vi "next order.vi"(8 "error in":errorcluster, 10 "Order":string, 11 "status":T1) -> (0 "error out":errorcluster, 3 "Order":string)   [LabVIEW 2015]
uses:
  status.ctl
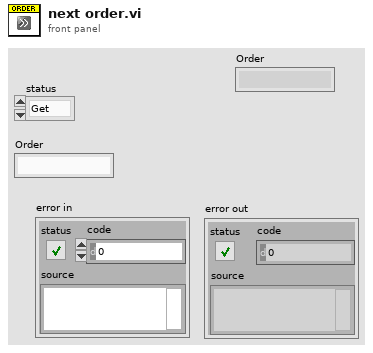
[diagram p1: front panel]
types:
  T1 = typedef "status.ctl" = enum16{"Get", "Set"}
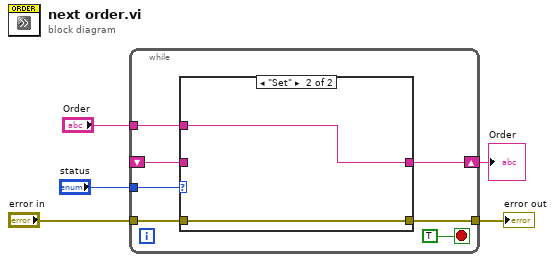
[diagram p0: block diagram]
diagram:
  n1 = while {
    shift-right: [w10] -> w1
    shift-left: _ -> [w8]
    tunnel: "status" -> [w11]
    tunnel: "Order" -> [w9]
    tunnel: "error in" -> [w7]
    tunnel: [w6] -> w2
    stop <- TRUE stop-if-true
    n2 = case shown="\"Set\"" w11 {
      tunnel: [w14 w16] -> w10
      tunnel: w9 -> [_ w16]
      tunnel: w8 -> [w14 _]
      tunnel: w7 -> [w13 w15]
      tunnel: [w13 w15] -> w6
      frame "Get", Default {
      }
      frame "Set" {
      }
    }
  }
  "error out" <- w2
  "Order" <- w1
